vi "Servo motor.vi"(8 "error in (no error)":errorcluster, 10 "Duty Cycle":dbl(knob)=0.5 scale=0.035..0.075) -> (0 "error out":errorcluster, 2 "Drop?":bool)   [LabVIEW 2015]
uses:
  <vilib>/myRIO/Instrument Drivers/Onboard IO/PWM/PWM.lvlib
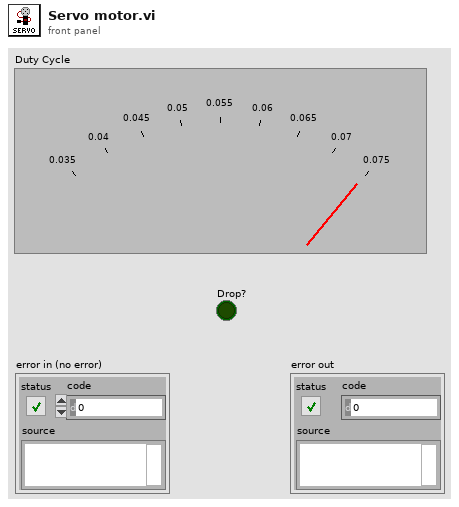
[diagram p1: front panel]
types:
  T1 = typedef "PWM.lvlib/PWM Reference.ctl" = cluster{"myRIO Reference":T2, "PWM Channels Enum":T6, "PWM Configuration":T7}
  T2 = typedef "myRIO Generic Hardware Reference.ctl" = cluster{"myRIO Model":T3, "myRIO Hardware Reference":T4}
  T3 = typedef "Hardware Version Enum.ctl" = enum16{"Unknown", "myRIO-1900", "myRIO-1950", "roboRIO", "NI ELVIS RIO CM"}
  T4 = typedef "myRIO v1.0 Reference.ctl" = cluster{"Generic FPGA Reference":T5, "Allow multiple opens":bool}
  T5 = typedef "Generic FPGA Reference.ctl" = refnum<k20>
  T6 = typedef "PWM Channels Enum.ctl" = enum16{"Not Connected", "C/PWM0", "C/PWM1", "A/PWM0", "A/PWM1", "A/PWM2", "B/PWM0", "B/PWM1", "B/PWM2", "PWM/PWM0", "PWM/PWM1", "PWM/PWM2", "PWM/PWM3", "PWM/PWM4", "PWM/PWM5", "PWM/PWM6", "PWM/PWM7", "PWM/PWM8", "PWM/PWM9"}
  T7 = typedef "PWM.lvlib/PWM Configuration.ctl" = cluster{"Frequency":dbl, "Duty Cycle":dbl}
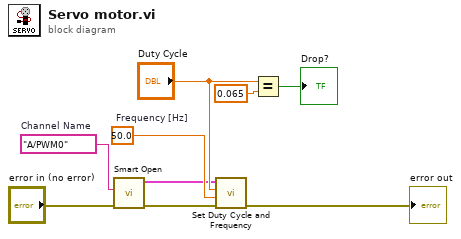
[diagram p0: block diagram]
diagram:
  w6 = 50.0  # Frequency [Hz]
  w7 = tag "A/PWM0"  # Channel Name
  n1 = call <vilib>:"Smart Open.vi"("error in (no error)"="error in (no error)", "Channel Name"=w7) -> ("error out"=w5:errorcluster, "PWM Ref Out"=w1:T1)  [unwired: 8 in]
  n2 = call <vilib>:"Set Duty Cycle and Frequency.vi"("error in (no error)"=w5, "Frequency [Hz]"=w6, "Duty Cycle"="Duty Cycle", "PWM Ref In"=w1) -> ("error out"=→"error out":errorcluster)  [unwired: 5 in, 1 out]
  n3 = Equal?(x="Duty Cycle", y=0.065) -> (x = y?=→"Drop?":bool)
